vi "Read_BSA_data_PWA.vi"(0 "GPIB Address":string="13", 7 "No of Check Bytes":i32, 9 "Bytes per block":i32, 11 "error in (no error)":errorcluster) -> (4 "transmission okay":bool, 8 "array of velocity data":u16[](array[numeric]), 15 "error out":errorcluster)   [LabVIEW 2010]
panel:
  out "Loop counter":i32
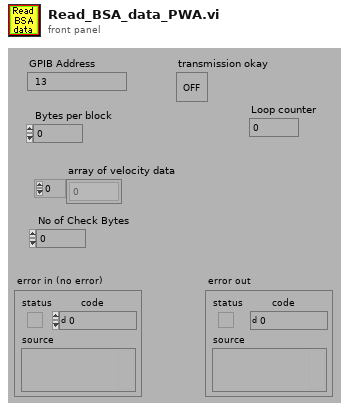
[diagram p1: front panel]
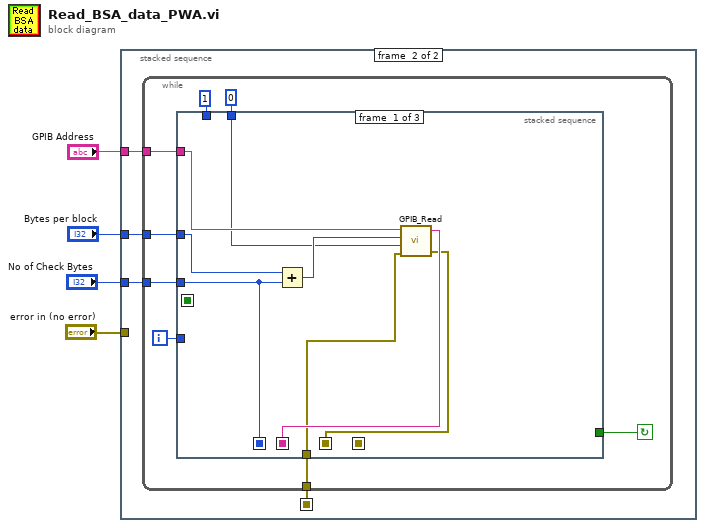
[diagram p0: block diagram]
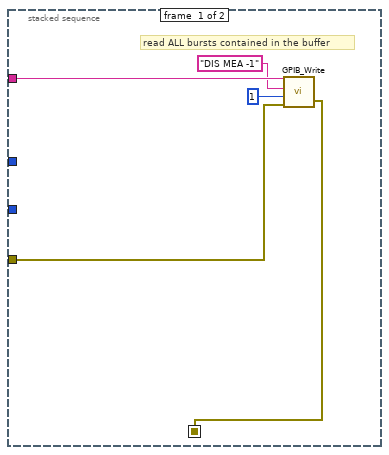
[diagram p2: hidden frame]
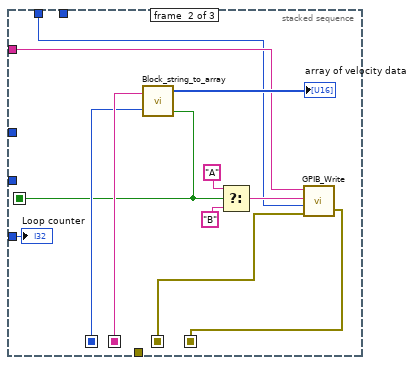
[diagram p3: hidden frame]
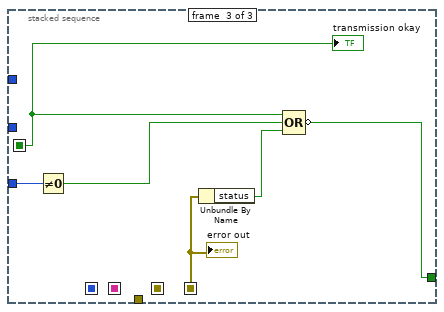
[diagram p4: hidden frame]
diagram:
  n1 = stacked-sequence {
    seq-local: [w6 _] -> [_ w12]
    tunnel: "GPIB Address" -> [w9 w13]
    tunnel: "Bytes per block" -> [_ w11]
    tunnel: "No of Check Bytes" -> [_ w10]
    tunnel: "error in (no error)" -> [w5 _]
    frame #0 {
      # "read ALL bursts contained in the buffer"
      n2 = call "GPIB_Write.vi"("address string"=w9, "data In"="DIS MEA -1", "mode (0)"=i16 1 ("mode"), "error in"=w5) -> ("error out"=w6:errorcluster)  [unwired: 1 in, 1 out]
    }
    frame #1 {
      n3 = while {
        tunnel: w12 -> [w16]
        tunnel: w13 -> [w21]
        tunnel: w11 -> [w15]
        tunnel: w10 -> [w14]
        i -> [w18]
        stop <- w17 continue-if-true
        n4 = stacked-sequence {
          seq-local: [w28 _ _] -> [_ w41 _]
          seq-local: [w22 _ _] -> [_ w40 _]
          seq-local: [_ w37 _] -> [_ _ w46]
          seq-local: [w24 _ _] -> [_ w31 _]
          seq-local: [_ w30 _] -> [_ _ w42]
          tunnel: w21 -> [w29 w33 _]
          tunnel: i16 0 ("Read mode") -> [w26 _ _]
          tunnel: 1 ("Write Mode") -> [_ w32 _]
          tunnel: w18 -> [_ w38 w47]
          tunnel: [_ _ w43] -> w17
          tunnel: w16 -> [w25 _ _]
          tunnel: w15 -> [w23 _ _]
          tunnel: w14 -> [w22 _ _]
          frame #0 {
            n5 = Add(x=w23, y=w22) -> (x+y=w27:i32)
            n6 = call "GPIB_Read.vi"("address string"=w29, "byte count"=w27, "mode (0)"=w26, "error in"=w25) -> ("data Out"=w28:string, "error out"=w24:errorcluster)  [unwired: 1 in, 1 out]
          }
          frame #1 {
            n7 = call "Block_string_to_array.vi"("transmitted string"=w41, "check size"=w40) -> ("array of velocity data"=→"array of velocity data":u16[], "transmission okay"=w37:bool)  [unwired: 1 out]
            n8 = Select(t="A", s=w37, f="B") -> (s? t:f=w34:string)
            n9 = call "GPIB_Write.vi"("address string"=w33, "data In"=w34, "mode (0)"=w32, "error in"=w31) -> ("error out"=w30:errorcluster)  [unwired: 1 in, 1 out]
            "Loop counter" <- w38
          }
          frame #2 {
            n10 = Not Equal To 0?(x=w47) -> (x != 0?=w45:bool)
            n11 = Unbundle By Name(w42) -> ("status"=w44:bool)
            n12 = Compound Arithmetic op=OR(w46, w45, w44) -> (invert w43:bool)
            "transmission okay" <- w46
            "error out" <- w42
          }
        }
      }
    }
  }
